vi "delay_time.vi"() -> ()   [LabVIEW 2011]
panel:
  in  "Delay Time":dbl
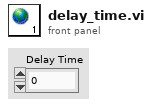
[diagram p1: front panel]
diagram:
